vi "Application Control View.vi"(10 "User Events in":refnum<class "User Events.lvclass">) -> ()   [LabVIEW 2016, in "HPMT_Views.lvlib"]
uses:
  HPMT_Views.lvlib
  User Events/User Events.lvclass
  Commands/Command Factory/Command Factory.lvclass
  User Events/User Events.lvclass/User Events.ctl
  Typedefs/StateTypes.ctl
  Typedefs/CommandTypes.ctl
  Typedefs/HPMT_Typedefs.lvlib
panel:
  in  "disableIsTrue":bool
  in  "enableIsTrue":bool
  in  "standbyIsTrue":bool
  in  "shutdownIsTrue":bool
  in  "startIsTrue":bool
types:
  T1 = typedef "HPMT_Typedefs.lvlib/Publish Data Events.ctl" = cluster{"State":refnum<user-event>, "ErrorCode":refnum<user-event>, "Scan Progress":refnum<user-event>, "All Test Status":refnum<user-event>, "ActuatorData":refnum<user-event>, "Test Settings":refnum<user-event>, "Stop Constant Query":refnum<user-event>}
  T2 = typedef "HPMT_Typedefs.lvlib/Subscribe Data Events.ctl" = cluster{"Command":refnum<user-event>}
  T3 = cluster{"Event Registration Refnum":refnum<event-registration>}
  T4 = typedef "HPMT_Typedefs.lvlib/StateTypes.ctl" = enum16{"Offline State", "Fault State", "Standby State", "Disabled State", "Enabled State", "Wait For User Input State", "Test Actuator State", "Manual State"}
  T5 = typedef "HPMT_Typedefs.lvlib/CommandTypes.ctl" = enum16{"Start", "Enable", "Disable", "Standby", "Shutdown", "Update", "Stiffness", "Move Steps", "Constant Query", "Stop Constant Query"}
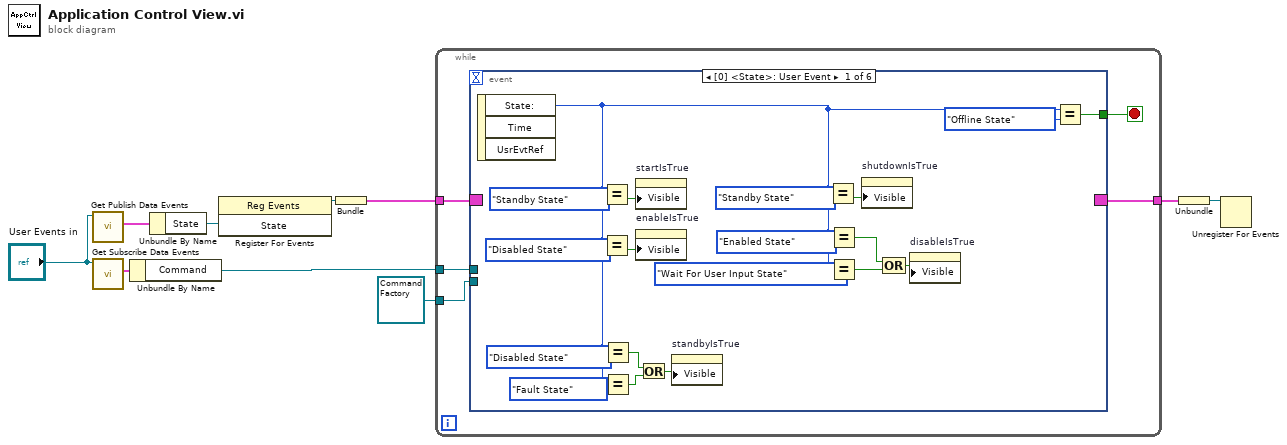
[diagram p0: block diagram]
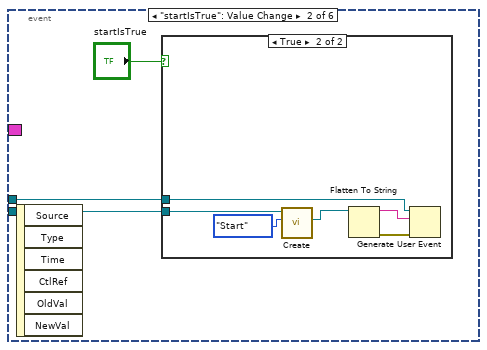
[diagram p2: hidden frame]
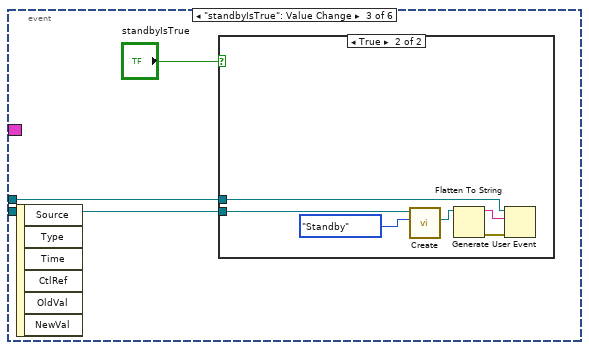
[diagram p4: hidden frame]
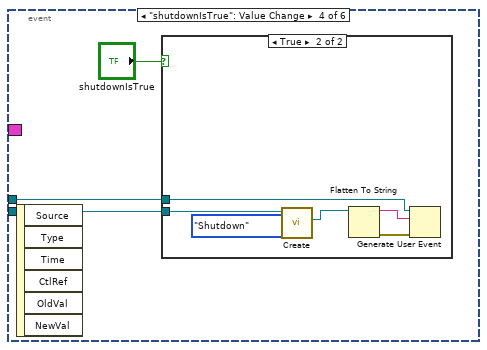
[diagram p6: hidden frame]
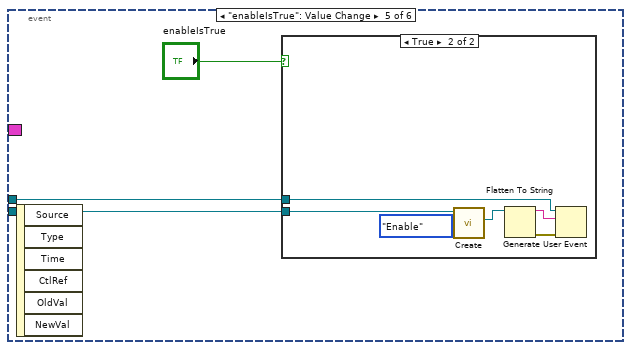
[diagram p8: hidden frame]
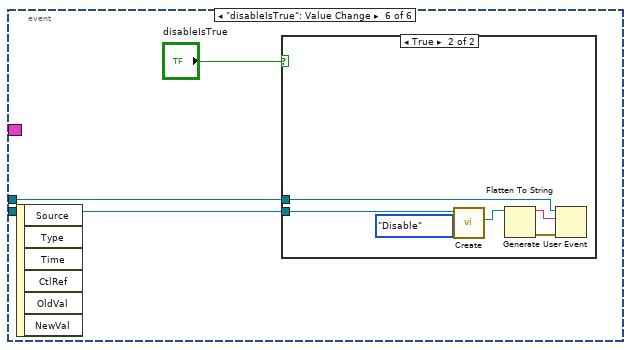
[diagram p10: hidden frame]
diagram:
  n1 = call "Get Publish Data Events.vi"("UserEvents in"="User Events in") -> ("Publish Data Events"=w7:T1)  [unwired: 9 in, 1 out]
  n2 = call "Get Subscribe Data Events.vi"("UserEvents in"="User Events in") -> ("Subscribe Data Events"=w8:T2)  [unwired: 9 in, 1 out]
  n3 = Unbundle By Name(w8) -> ("Command"=w5:refnum<user-event>)
  n4 = Unbundle By Name(w7) -> ("State"=w9:refnum<user-event>)
  n5 = register-events(w9) -> (reference out=w10:refnum<event-registration>)  [unwired: 2 in, 1 out]
  n6 = Bundle("Event Registration Refnum"=w10) -> (w6:T3)  [unwired: 1 in]
  n7 = while {
    tunnel: w6 -> [w15]
    tunnel: w5 -> [w14]
    tunnel: [w13] -> w4
    tunnel: refnum<class "Command Factory.lvclass"> refnum ("CommandFactory.lvclass") -> [w11]
    stop <- w12 stop-if-true
    n8 = event shown="[0] <State>: User Event" {
      selector: w15 -> [_ _ _ _ _ _]
      dyn-events: [_ _ _ _ _ _] -> w13
      timeout: _ -> [_ _ _ _ _ _]
      tunnel: w14 -> [_ w37 w45 w54 w63 w72]
      tunnel: [w33 _ _ _ _ _] -> w12
      tunnel: w11 -> [_ w36 w46 w55 w64 w73]
      event User Event {
        n9 = event-data() -> ("State:"=w16:T4)  [unwired: 1 in, 2 out]
        n10 = Equal?(x=w16, y=StateTypes."Standby State") -> (x = y?=w31:bool)
        n11 = Equal?(x=w16, y=StateTypes."Disabled State") -> (x = y?=w30:bool)
        n12 = Equal?(x=w16, y=StateTypes."Disabled State") -> (x = y?=w25:bool)
        n13 = Equal?(x=w16, y=StateTypes."Fault State") -> (x = y?=w26:bool)
        n14 = property on="startIsTrue" class="Bool"("Visible"=w31) -> ()  [unwired: 2 in, 2 out]
        n15 = property on="enableIsTrue" class="Bool"("Visible"=w30) -> ()  [unwired: 2 in, 2 out]
        n16 = Or(x=w25, y=w26) -> (x .or. y?=w24:bool)
        n17 = property on="standbyIsTrue" class="Bool"("Visible"=w24) -> ()  [unwired: 2 in, 2 out]
        n18 = Equal?(x=w16, y=StateTypes."Standby State") -> (x = y?=w23:bool)
        n19 = Equal?(x=w16, y=StateTypes."Enabled State") -> (x = y?=w18:bool)
        n20 = Equal?(x=w16, y=StateTypes."Wait For User Input State") -> (x = y?=w19:bool)
        n21 = property on="shutdownIsTrue" class="Bool"("Visible"=w23) -> ()  [unwired: 2 in, 2 out]
        n22 = Compound Arithmetic op=OR(w18, w19) -> (w17:bool)
        n23 = property on="disableIsTrue" class="Bool"("Visible"=w17) -> ()  [unwired: 2 in, 2 out]
        n24 = Equal?(x=w16, y=StateTypes."Offline State") -> (x = y?=w33:bool)
      }
      event "startIsTrue": Value Change {
        n25 = event-data() -> ()  [unwired: 1 in, 6 out]
        n26 = case shown="True" "startIsTrue" {
          tunnel: w36 -> [_ w43]
          tunnel: w37 -> [_ w39]
          frame False {
          }
          frame True {
            n27 = call-dynamic "Create.vi"("Command Types"=CommandTypes."Start" ("Command"), "Command Factory in"=w43) -> ("Command"=w38:refnum<class "Command.lvclass">)  [unwired: 7 in, 2 out]
            n28 = Flatten To String(anything=w38) -> (data string=w40:string, error out=w41:errorcluster)  [unwired: 3 in, 1 out]
            n29 = Generate User Event(user event=w39, event data cluster=w40, error in=w41) -> ()  [unwired: 1 in, 2 out]
          }
        }
      }
      event "standbyIsTrue": Value Change {
        n30 = event-data() -> ()  [unwired: 1 in, 6 out]
        n31 = case shown="True" "standbyIsTrue" {
          tunnel: w46 -> [_ w52]
          tunnel: w45 -> [_ w48]
          frame False {
          }
          frame True {
            n32 = call-dynamic "Create.vi"("Command Types"=CommandTypes."Standby" ("Command"), "Command Factory in"=w52) -> ("Command"=w47:refnum<class "Command.lvclass">)  [unwired: 7 in, 2 out]
            n33 = Flatten To String(anything=w47) -> (data string=w49:string, error out=w50:errorcluster)  [unwired: 3 in, 1 out]
            n34 = Generate User Event(user event=w48, event data cluster=w49, error in=w50) -> ()  [unwired: 1 in, 2 out]
          }
        }
      }
      event "shutdownIsTrue": Value Change {
        n35 = event-data() -> ()  [unwired: 1 in, 6 out]
        n36 = case shown="True" "shutdownIsTrue" {
          tunnel: w55 -> [_ w61]
          tunnel: w54 -> [_ w57]
          frame False {
          }
          frame True {
            n37 = call-dynamic "Create.vi"("Command Types"=CommandTypes."Shutdown" ("Command"), "Command Factory in"=w61) -> ("Command"=w56:refnum<class "Command.lvclass">)  [unwired: 7 in, 2 out]
            n38 = Flatten To String(anything=w56) -> (data string=w58:string, error out=w59:errorcluster)  [unwired: 3 in, 1 out]
            n39 = Generate User Event(user event=w57, event data cluster=w58, error in=w59) -> ()  [unwired: 1 in, 2 out]
          }
        }
      }
      event "enableIsTrue": Value Change {
        n40 = event-data() -> ()  [unwired: 1 in, 6 out]
        n41 = case shown="True" "enableIsTrue" {
          tunnel: w64 -> [_ w70]
          tunnel: w63 -> [_ w66]
          frame False {
          }
          frame True {
            n42 = call-dynamic "Create.vi"("Command Types"=CommandTypes."Enable" ("Command"), "Command Factory in"=w70) -> ("Command"=w65:refnum<class "Command.lvclass">)  [unwired: 7 in, 2 out]
            n43 = Flatten To String(anything=w65) -> (data string=w67:string, error out=w68:errorcluster)  [unwired: 3 in, 1 out]
            n44 = Generate User Event(user event=w66, event data cluster=w67, error in=w68) -> ()  [unwired: 1 in, 2 out]
          }
        }
      }
      event "disableIsTrue": Value Change {
        n45 = event-data() -> ()  [unwired: 1 in, 6 out]
        n46 = case shown="True" "disableIsTrue" {
          tunnel: w73 -> [_ w79]
          tunnel: w72 -> [_ w75]
          frame False {
          }
          frame True {
            n47 = call-dynamic "Create.vi"("Command Types"=CommandTypes."Disable" ("Command"), "Command Factory in"=w79) -> ("Command"=w74:refnum<class "Command.lvclass">)  [unwired: 7 in, 2 out]
            n48 = Flatten To String(anything=w74) -> (data string=w76:string, error out=w77:errorcluster)  [unwired: 3 in, 1 out]
            n49 = Generate User Event(user event=w75, event data cluster=w76, error in=w77) -> ()  [unwired: 1 in, 2 out]
          }
        }
      }
    }
  }
  n50 = Unbundle(w4) -> ("Event Registration Refnum"=w3:refnum<event-registration>)
  n51 = Unregister For Events(event registration refnum=w3) -> ()  [unwired: 1 in, 1 out]
